vi "CreaInformeExcel.vi"(0 "UnidadesF":refnum<vi>, 1 "ValorParoDesplazamiento":dbl, 2 "TipusAssaig":string, 3 "ActivaParoDefor":bool, 4 "VelocidadEnsayo":dbl, 5 "ArraiMostresxProva":dbl[](array[numeric]), 6 "Nom Assaig":string, 7 "Precarga":bool, 8 "NºTests":u8, 9 "ValorPrecarga":dbl, 10 "UnidadesD":refnum<vi>, 11 "ActivaParoRotura":bool, 12 "TablaFinal":dbl[][](array[numeric]), 13 "ValorParoRotura":dbl) -> (14 "status":bool)   [LabVIEW 2017]
uses:
  <vilib>/addons/_office/excel.llb/Excel Easy Table (num).vi
  <vilib>/addons/_office/excel.llb/Excel Easy Table (str).vi
  <vilib>/Utility/NIReport.llb/NI_report.lvclass
  <vilib>/addons/_office/NI_ReportGenerationToolkit.lvlib
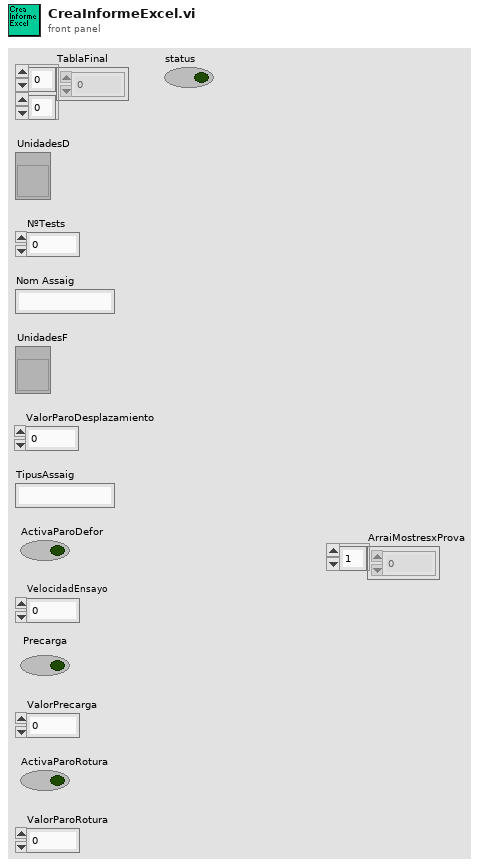
[diagram p1: front panel]
types:
  T1 = enum16{"maximized", "minimized", "normal", "no change"}
  T2 = enum16{"Standard Report", "HTML", "Word", "Excel"}
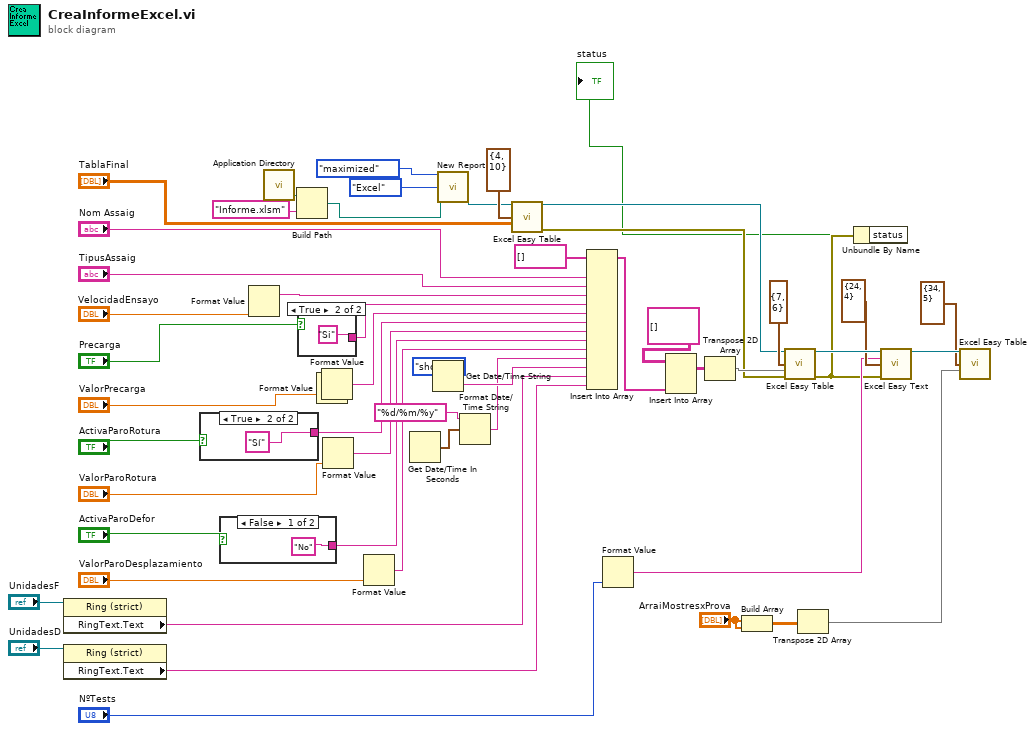
[diagram p0: block diagram]
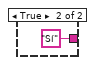
[diagram p2: hidden frame]
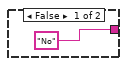
[diagram p3: hidden frame]
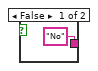
[diagram p4: hidden frame]
diagram:
  n1 = property on="Property Node" class="Ring (strict)"(reference="UnidadesF") -> ("RingText.Text"=w11:string)  [unwired: 1 in, 2 out]
  n2 = property on="Property Node" class="Ring (strict)"(reference="UnidadesD") -> ("RingText.Text"=w12:string)  [unwired: 1 in, 2 out]
  n3 = case shown="True" "ActivaParoRotura" {
    tunnel: ["No" "Sí"] -> w41
    frame False {
    }
    frame True {
    }
  }
  n4 = case shown="False" "ActivaParoDefor" {
    tunnel: ["No" "Sí"] -> w43
    frame False {
    }
    frame True {
    }
  }
  n5 = Format Value(value (0)="VelocidadEnsayo") -> (output string=w33:string)  [unwired: 2 in]
  n6 = call <vilib>:"Application Directory.vi"() -> ("Application Directory"=w19:path)
  n7 = Build Path(base path=w19, name or relative path="Informe.xlsm") -> (appended path=w21:path)
  n8 = case shown="True" "Precarga" {
    tunnel: ["No" "Si"] -> w38
    frame False {
    }
    frame True {
    }
  }
  n9 = Format Value() -> ()  [unwired: 3 in, 1 out]
  n10 = Format Value(value (0)="ValorPrecarga") -> (output string=w40:string)  [unwired: 2 in]
  n11 = Format Value(value (0)="ValorParoRotura") -> (output string=w42:string)  [unwired: 2 in]
  n12 = Format Value(value (0)="ValorParoDesplazamiento") -> (output string=w44:string)  [unwired: 2 in]
  n13 = Get Date/Time In Seconds() -> (seconds since 1Jan1904=w2:timestamp)
  n14 = Get Date/Time String(date format (0)=enum16{"short", "long", "abbreviated"}."short") -> (time string=w10:string)  [unwired: 2 in, 1 out]
  n15 = call <vilib>:"New Report.vi"("window state (normal)"=T1."maximized", "report type"=T2."Excel", "template (empty)"=w21) -> ("report out"=w23:refnum<class "NI_report.lvclass">)  [unwired: 11 in, 1 out]
  n16 = Format Date/Time String(time format string (%c)="%d/%m/%y", seconds (now)=w2) -> (date/time string=w1:string)  [unwired: 1 in]
  n17 = call-poly <vilib>:"Excel Easy Table.vi"("report in"=w23, "start (0, 0)"=cluster{"row":i32, "column":i32} {"row"=4, "column"=10}, "text data"="TablaFinal") -> ("report out"=w28:refnum<class "NI_report.lvclass">, "error out"=w29:errorcluster)  [unwired: 8 in, 3 out]
  n18 = Insert Into Array(array=string[] [] ("new element/subarray"), new element #1="Nom Assaig", new element #2="TipusAssaig", new element #3=w33, new element #4=w38, new element #5=w40, new element #6=w41, new element #7=w42, new element #8=w43, new element #9=w44, new element #10=w1, new element #11=w10, new element #12=w11, new element #13=w12) -> (w35:string[])  [unwired: 1 in]
  n19 = Format Value(value (0)="NºTests") -> (output string=w49:string)  [unwired: 2 in]
  n20 = Insert Into Array(array=string[][] [] ("text data"), new element=w35) -> (w37:string[][])  [unwired: 2 in]
  n21 = Transpose 2D Array(2D array=w37) -> (transposed array=w36:string[][])
  n22 = Build Array("ArraiMostresxProva", "ArraiMostresxProva") -> (w6:dbl[][])
  n23 = call-poly <vilib>:"Excel Easy Table.vi"("report in"=w28, "start (0, 0)"=cluster{"row":i32, "column":i32} {"row"=7, "column"=6}, "text data"=w36, "error in (no error)"=w29) -> ("report out"=w51:refnum<class "NI_report.lvclass">, "error out"=w47:errorcluster)  [unwired: 7 in, 3 out]
  n24 = Transpose 2D Array(2D array=w6) -> (transposed array=w5:dbl[][])
  n25 = Unbundle By Name(w47) -> ("status"=→"status":bool)
  n26 = call <vilib>:"Excel Easy Text.vi"("report in"=w51, "text"=w49, "start (-1, -1)"=cluster{"row":i32, "column":i32} {"row"=24, "column"=4} ("start (0, 0)"), "error in (no error)"=w47) -> ("report out"=w9:refnum<class "NI_report.lvclass">)  [unwired: 7 in, 4 out]
  n27 = call-poly <vilib>:"Excel Easy Table.vi"("report in"=w9, "start (0, 0)"=cluster{"row":i32, "column":i32} {"row"=34, "column"=5}, "text data"=w5) -> ()  [unwired: 8 in, 5 out]
